vi "Beat Demo.vi"() -> ()   [LabVIEW 2020]
uses:
  <vilib>/measure/NI_MABase.lvlib
panel:
  out "Signal 1+2Spectrum":cluster{"f0":dbl, "df":dbl, "magnitude":dbl[]}[](graph)
  out "Signal 2 Spectrum":cluster{"f0":dbl, "df":dbl, "magnitude":dbl[]}[](graph)
  out "Signal 1 Spectrum":cluster{"f0":dbl, "df":dbl, "magnitude":dbl[]}[](graph)
  in  "Stop Button":bool
  out "Signals 1+2":waveform(dbl)(graph)={"t0"=timestamp(0 s since 1904-01-01), "dt"=0.02, "Y"=array[2000 elements]}
  out "Signal 2":waveform(dbl)(graph)={"t0"=timestamp(0 s since 1904-01-01), "dt"=0.02, "Y"=array[2000 elements]}
  out "Signal 1":waveform(dbl)(graph)={"t0"=timestamp(0 s since 1904-01-01), "dt"=0.02, "Y"=array[2000 elements]}
  in  "Input Signals":cluster{"Frequency":dbl, "Amplitude":dbl}[](array[cluster])=[{"Frequency"=1.0, "Amplitude"=1.0}, {"Frequency"=1.1000000000000003, "Amplitude"=1.0}] {"Amplitude" step=0.1 format="%.1g"; "Frequency" step=0.05 format="%.2g"}
  # "Beat Demo"
  # "McClellan et al., \nDSP First\nCh. 3-2 Beat Notes"
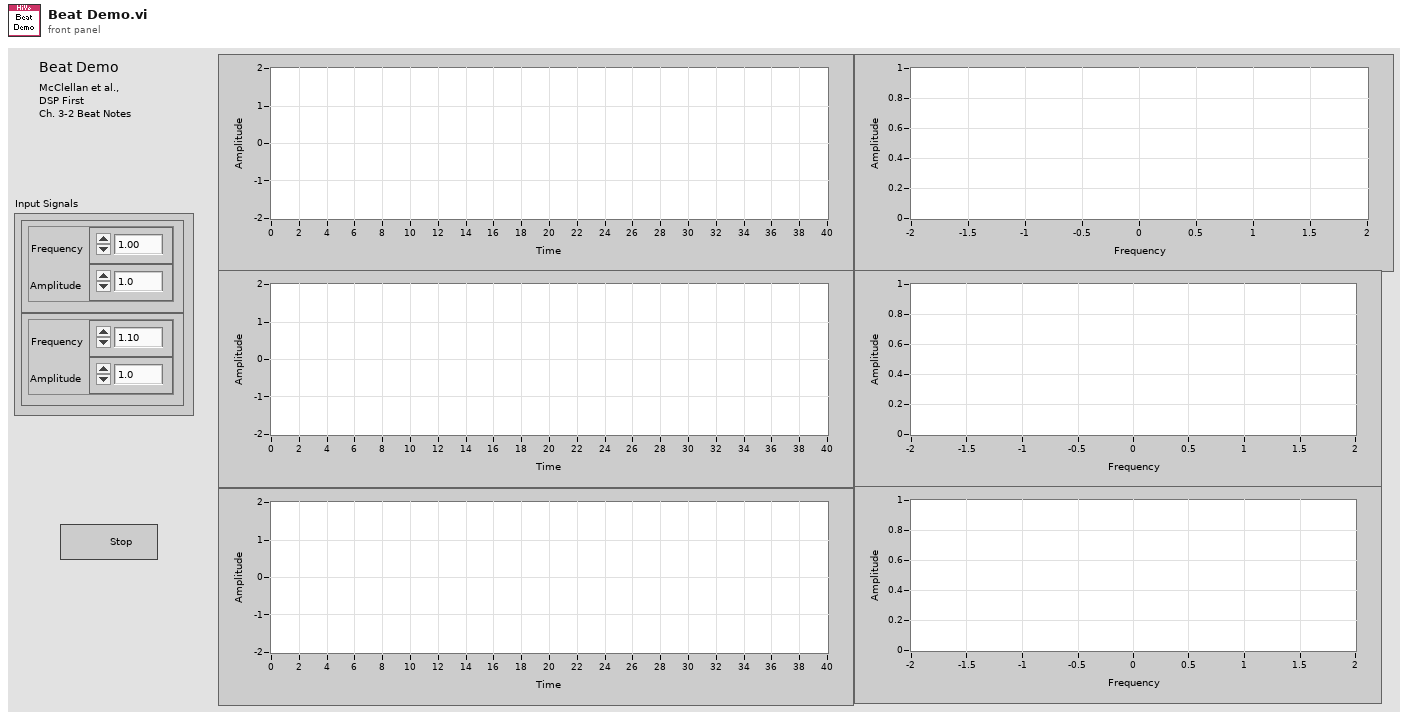
[diagram p1: front panel]
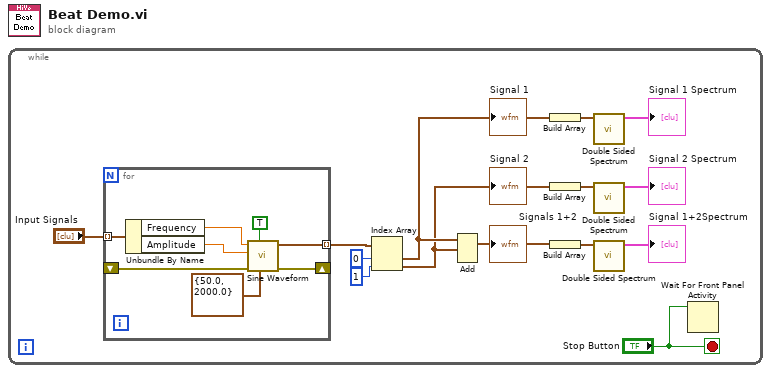
[diagram p0: block diagram]
diagram:
  n1 = while {
    stop <- "Stop Button" stop-if-true
    n2 = for {
      tunnel: "Input Signals" -> [w22] mode=indexing
      shift-right: [w19] -> _
      shift-left: _ -> [w18]
      tunnel: [w17] -> w13 mode=indexing
      n3 = Unbundle By Name(w22) -> ("Frequency"=w20:dbl, "Amplitude"=w21:dbl)
      n4 = call <vilib>:"Sine Waveform.vi"("sampling info"=cluster{"Fs":dbl, "#s":dbl} {"Fs"=50.0, "#s"=2000.0}, "reset signal"=TRUE, "error in (no error)"=w18, "amplitude"=w21, "frequency"=w20) -> ("error out"=w19:errorcluster, "signal out"=w17:waveform(dbl))  [unwired: 5 in]
    }
    n5 = Index Array(array=w13, index #1=0 ("index"), index #2=1 ("index")) -> (element #1=w8:waveform(dbl), element #2=w5:waveform(dbl))
    "Signal 1" <- w8
    "Signal 2" <- w5
    n6 = Add(1:w5, 2:w8) -> (0:w4:waveform(dbl))  [unwired: 1 in, 1 out]
    "Signals 1+2" <- w4
    n7 = Build Array(w8) -> (w3:waveform(dbl)[])
    n8 = Build Array(w5) -> (w2:waveform(dbl)[])
    n9 = Build Array(w4) -> (w1:waveform(dbl)[])
    n10 = call "Double Sided Spectrum.vi"("Signals In"=w3) -> ("Double Sided Spectra"=→"Signal 1 Spectrum":cluster{"f0":dbl, "df":dbl, "magnitude":dbl[]}[])  [unwired: 9 in, 1 out]
    n11 = call "Double Sided Spectrum.vi"("Signals In"=w2) -> ("Double Sided Spectra"=→"Signal 2 Spectrum":cluster{"f0":dbl, "df":dbl, "magnitude":dbl[]}[])  [unwired: 9 in, 1 out]
    n12 = call "Double Sided Spectrum.vi"("Signals In"=w1) -> ("Double Sided Spectra"=→"Signal 1+2Spectrum":cluster{"f0":dbl, "df":dbl, "magnitude":dbl[]}[])  [unwired: 9 in, 1 out]
    n13 = Wait For Front Panel Activity(3:"Stop Button") -> ()  [unwired: 2 in, 1 out]
  }
